vi "Read Board Status.vi"(0 "Session Handle in":T1, 11 "error in (no error)":errorcluster) -> (4 "Session Handle out":T1, 6 "Ready?":bool, 15 "error out":errorcluster)   [LabVIEW 2015, in "PAS.lvclass"]
uses:
  PAS.lvclass
  Typedefs/Session Handle.ctl
panel:
  out "Board Reset Status":u8
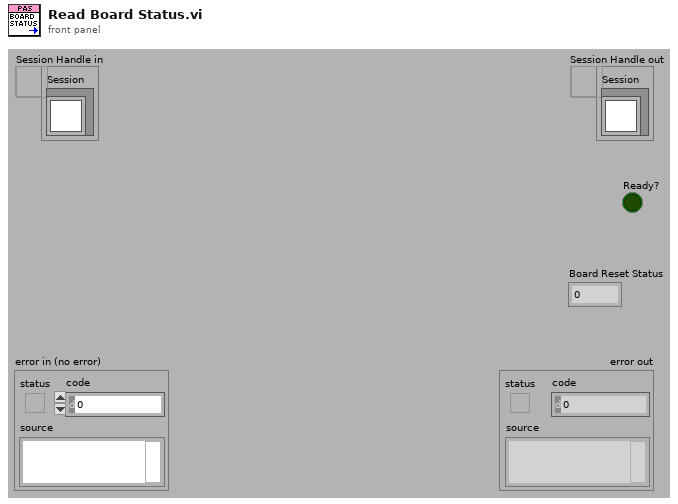
[diagram p1: front panel]
types:
  T1 = typedef "PAS.lvclass/Session Handle.ctl" = refnum<data-value>
  T2 = typedef "XNET Frame CAN.ctl" = cluster{"timestamp":timestamp, "payload":u8[], "identifier":u32, "type":T3, "extended?":bool, "echo?":bool}
  T3 = typedef "XNET Frame Type CAN.ctl" = u8
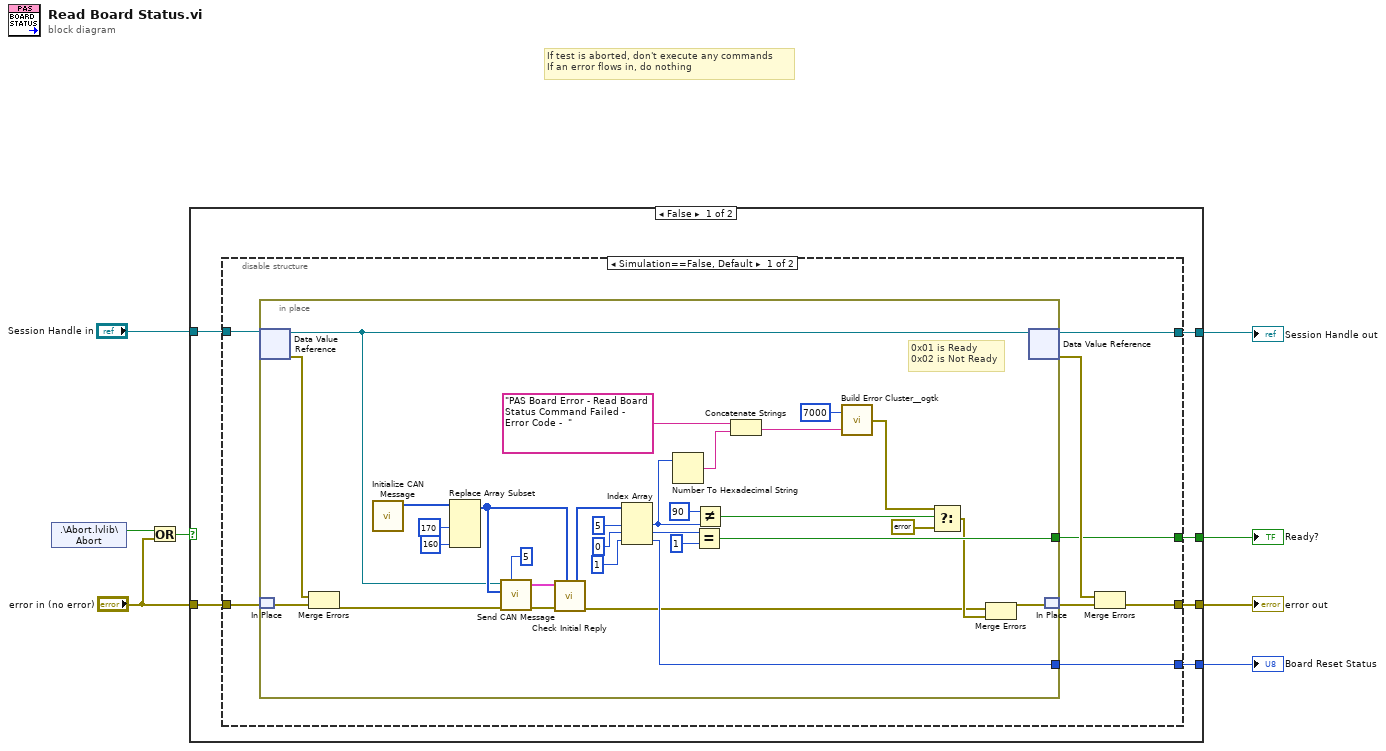
[diagram p0: block diagram]
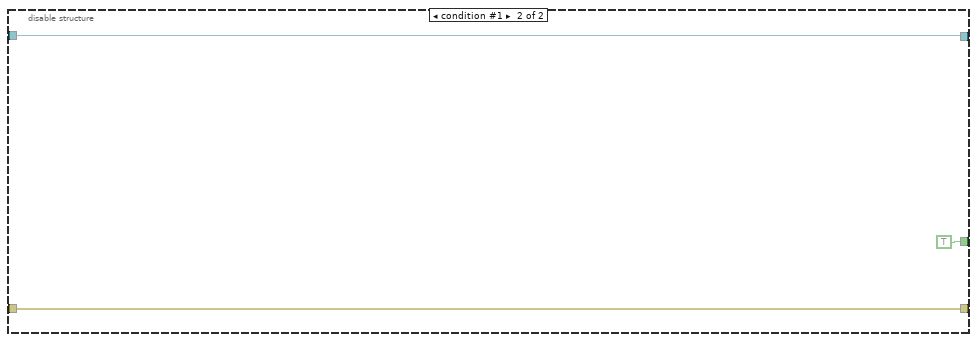
[diagram p2: hidden frame]
diagram:
  # "If test is aborted, don't execute any commands\nIf an error flows in, do nothing"
  n1 = shared-variable ".\\Abort.lvlib\\Abort"() -> (w5:bool)  [unwired: 1 in, 1 out]
  n2 = Or(x=w5, y="error in (no error)") -> (x .or. y?=w3:bool)
  n3 = case shown="False" w3 {
    tunnel: [w14 w58] -> w7
    tunnel: [w13 w57] -> w6
    tunnel: "Session Handle in" -> [w12 w58]
    tunnel: "error in (no error)" -> [w11 w57]
    tunnel: [w10 _] -> w2
    tunnel: [w9 _] -> w1
    frame False {
      n4 = disable-structure shown="Simulation==False, Default" {
        disable-tunnel: [w22 w56] -> w14
        disable-tunnel: [w19 w55] -> w13
        disable-tunnel: w12 -> [w18 w56]
        disable-tunnel: w11 -> [w17 w55]
        disable-tunnel: [w16 TRUE] -> w10
        disable-tunnel: [w15 _] -> w9
        frame condition #0 (active) {
          n5 = in-place {
            in-place-border: [w32] -> w16
            in-place-border: [w26] -> w15
            # "0x01 is Ready\n0x02 is Not Ready"
            n6 = in-place-dvr #1(w18) -> (w44:refnum<class "PAS.lvclass">, w48:errorcluster)
            n7 = in-place-match #2(w17) -> (w47:errorcluster)
            n8 = Merge Errors(w48, w47) -> (w46:errorcluster)
            n9 = call "Initialize CAN Message.vi"() -> ("Initial Payload"=w50:u8[])  [unwired: 11 in]
            n10 = Replace Array Subset(array=w50, new element #1=u8 170 ("new element/subarray"), new element #2=u8 160 ("new element/subarray")) -> (w45:u8[])  [unwired: 2 in]
            n11 = call "Send CAN Message.vi"("Number of Retries"=5, "error in (no error)"=w46, "payload"=w45, "Pas In"=w44) -> ("error out"=w24:errorcluster, "Reply"=w42:T2[])  [unwired: 5 in, 1 out]
            n12 = call "Check Initial Reply.vi"("Write Message"=w45, "error in (no error)"=w24, "Reply"=w42) -> ("error out"=w23:errorcluster, "Data Packet"=w49:u8[])  [unwired: 5 in, 2 out]
            n13 = Index Array(array=w49, index #1=5 ("index"), index #2=0 ("index"), index #3=1 ("index")) -> (element #1=w30:u8, element #2=w34:u8, element #3=w26:u8)
            n14 = Number To Hexadecimal String(2:w30) -> (0:w29:string)  [unwired: 1 in]
            n15 = Equal?(x=w34, y=u8 1) -> (x = y?=w32:bool)
            n16 = Not Equal?(x=u8 90 ("new element/subarray"), y=w30) -> (x != y?=w38:bool)
            n17 = Concatenate Strings("PAS Board Error - Read Board Status Command Failed - Error Code -  " ("string"), w29) -> (w28:string)
            n18 = call <userlib>:"Build Error Cluster__ogtk.vi"("String to Prepend to source (\"\")"=w28, "code"=7000) -> ("error out"=w40:errorcluster)
            n19 = Select(t=w40, s=w38, f=errorcluster {"status"=FALSE, "code"=0, "source"=""}) -> (s? t:f=w25:errorcluster)
            n20 = Merge Errors(w23, w25) -> (w51:errorcluster)
            n21 = in-place-dvr #1(w44) -> (w22:T1, w20:errorcluster)
            n22 = in-place-match #2(w51) -> (w21:errorcluster)
          }
          n23 = Merge Errors(w20, w21) -> (w19:errorcluster)
        }
        frame condition #1 {
        }
      }
    }
    frame True {
    }
  }
  "Session Handle out" <- w7
  "error out" <- w6
  "Ready?" <- w2
  "Board Reset Status" <- w1
